vi "Obtain Semaphore Reference.vi"(4 "error in (no error)":errorcluster, 5 "create if not found (T)":bool=TRUE, 6 "size (1)":i32=1, 7 "name (unnamed)":string) -> (0 "error out":errorcluster, 1 "created new":bool, 3 "semaphore":T1)   [LabVIEW 2020]
doc: "Obtains a reference to an existing semaphore or creates a new semaphore and returns a reference to that semaphore."
uses:
  Semaphore Refnum Core.ctl
  GetNamedSemaphorePrefix.vi
panel:
  in  "Size Mismatch\nWarning":string="<err>You specified a named semaphore that already exists, but the existing semaphore has a different size than the one you specified. LabVIEW returned a reference to the existing semaphore but did not resize the semaphore."
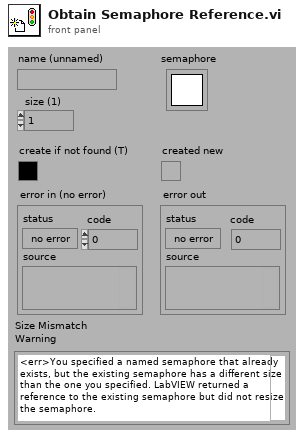
[diagram p1: front panel]
types:
  T1 = typedef "Semaphore RefNum" = refnum<k1>
  T2 = typedef "Semaphore Refnum Core.ctl" = refnum<k1>
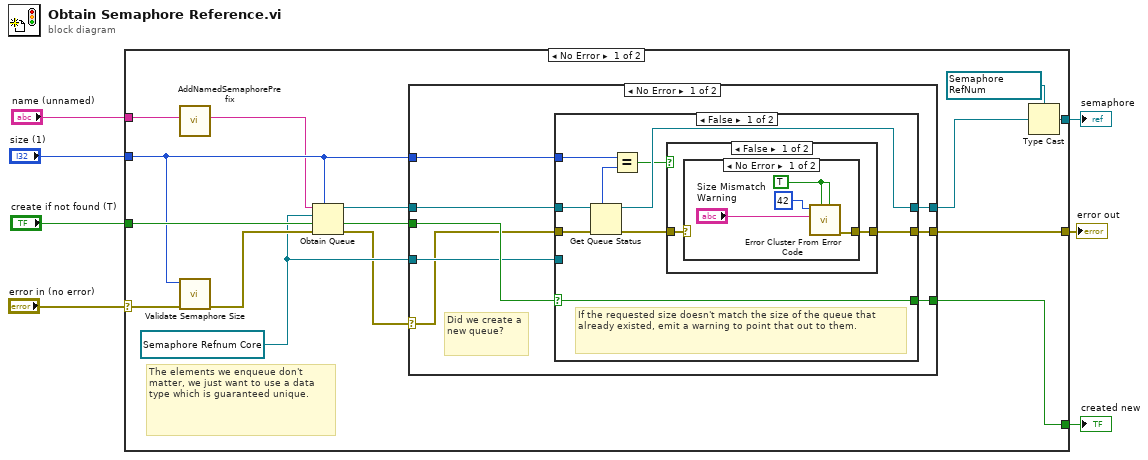
[diagram p0: block diagram]
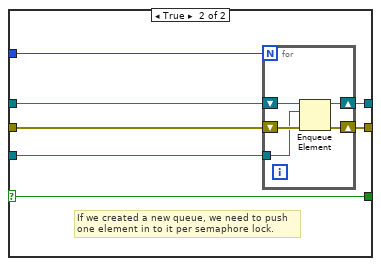
[diagram p4: hidden frame]
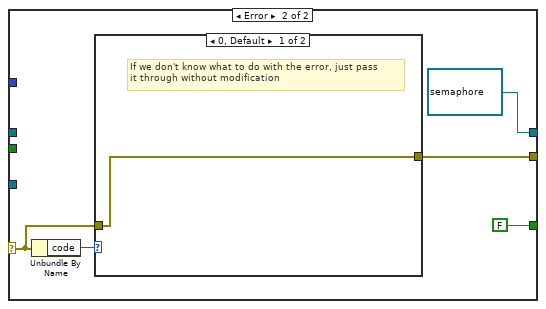
[diagram p5: hidden frame]
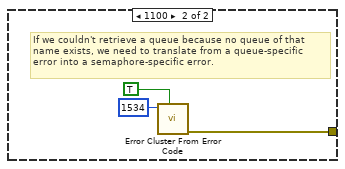
[diagram p6: hidden frame]
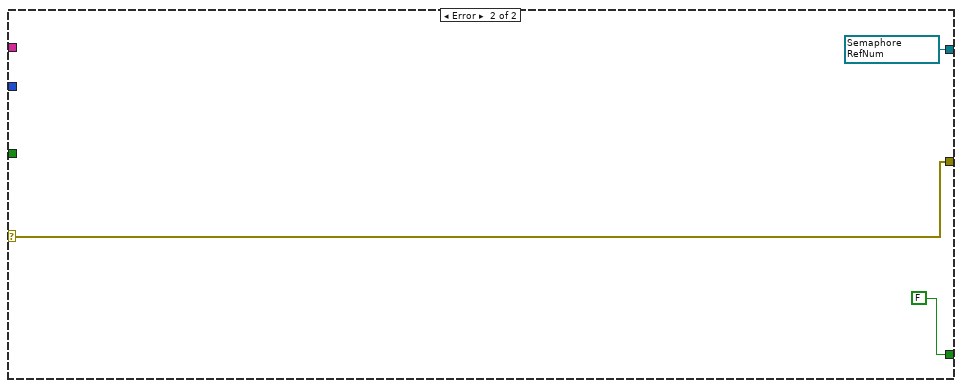
[diagram p7: hidden frame]
diagram:
  n1 = case shown="No Error" "error in (no error)" {
    selector: "error in (no error)" -> [w13 w70]
    tunnel: "create if not found (T)" -> [w21 _]
    tunnel: "name (unnamed)" -> [w9 _]
    tunnel: [w20 w69] -> w6
    tunnel: [w17 w70] -> w5
    tunnel: [w10 FALSE ("created new?")] -> w4
    tunnel: "size (1)" -> [w15 _]
    frame No Error {
      w14 = T2 refnum items=["Semaphore Core"] ("semaphore")
      w19 = T1 refnum items=["semaphore"] ("semaphore")
      # "The elements we enqueue don't matter, we just want to use a data type which is guaranteed unique."
      n2 = call "AddNamedSemaphorePrefix.vi"("String In"=w9) -> ("String Out"=w8:string)  [unwired: 10 out]
      n3 = call "Validate Semaphore Size.vi"("error in (no error)"=w13, "size (1)"=w15) -> ("error out"=w16:errorcluster)  [unwired: 5 out]
      n4 = Obtain Queue(max queue size (-1, unlimited)=w15, name (unnamed)=w8, element data type=w14, create if not found? (T)=w21, error in (no error)=w16) -> (queue out=w22:refnum<queue>, created new?=w11:bool, error out=w12:errorcluster)
      n5 = case shown="No Error" w12 {
        selector: w12 -> [w24 w62]
        tunnel: w22 -> [w30 _]
        tunnel: [w29 w60] -> w18
        tunnel: [w28 w61] -> w17
        tunnel: w11 -> [w27 _]
        tunnel: w15 -> [w26 _]
        tunnel: w14 -> [w25 _]
        tunnel: [w23 FALSE] -> w10
        frame No Error {
          # "Did we create a new queue?"
          n6 = case shown="False" w27 {
            selector: w27 -> [w31 w48]
            tunnel: w30 -> [w38 w54]
            tunnel: w24 -> [w39 w53]
            tunnel: w25 -> [_ w52]
            tunnel: w26 -> [w36 w51]
            tunnel: [w33 w50] -> w29
            tunnel: [w34 w49] -> w28
            tunnel: [w31 w48] -> w23
            frame False {
              # "If the requested size doesn't match the size of the queue that already existed, emit a warning to point that out to them."
              n7 = Get Queue Status(queue=w38, error in (no error)=w39) -> (queue out=w33:refnum<queue>, max queue size=w37:i32, error out=w35:errorcluster)  [unwired: 6 out]
              n8 = Equal?(x=w36, y=w37) -> (x = y?=w32:bool)
              n9 = case shown="False" w32 {
                tunnel: w35 -> [w41 w47]
                tunnel: [w40 w47] -> w34
                frame False {
                  n10 = case shown="No Error" w41 {
                    selector: w41 -> [_ w46]
                    tunnel: [w45 w46] -> w40
                    frame No Error {
                      w42 = TRUE ("show call chain? (False)")
                      n11 = call "Error Cluster From Error Code.vi"("is warning? (False)"=w42, "show call chain? (False)"=w42, "error message (\"\")"="Size Mismatch\nWarning", "error code (0)"=42) -> ("error out"=w45:errorcluster)  [unwired: 1 in, 4 out]
                    }
                    frame Error {
                    }
                  }
                }
                frame True {
                }
              }
            }
            frame True {
              # "If we created a new queue, we need to push one element in to it per semaphore lock."
              n12 = for {
                N: w51 -> [_]
                tunnel: w52 -> [w57]
                shift-right: [w56] -> w49
                shift-left: w53 -> [w58]
                shift-right: [w55] -> w50
                shift-left: w54 -> [w59]
                n13 = Enqueue Element(queue=w59, element=w57, error in (no error)=w58) -> (queue out=w55:refnum<queue>, error out=w56:errorcluster)  [unwired: 2 out]
              }
            }
          }
        }
        frame Error {
          w60 = refnum<queue> refnum items=["Semaphore Core"] ("queue out")
          n14 = Unbundle By Name(w62) -> ("code"=w63:i32)
          n15 = case shown="0, Default" w63 {
            tunnel: w62 -> [w65 _]
            tunnel: [w65 w68] -> w61
            frame 0, Default {
              # "If we don't know what to do with the error, just pass\nit through without modification"
            }
            frame 1100 {
              # "If we couldn't retrieve a queue because no queue of that\nname exists, we need to translate from a queue-specific\nerror into a semaphore-specific error."
              n16 = call "Error Cluster From Error Code.vi"("show call chain? (False)"=TRUE, "error code (0)"=1534) -> ("error out"=w68:errorcluster)  [unwired: 1 in, 6 out]
            }
          }
        }
      }
      n17 = Type Cast(type=w19, x=w18) -> (*(type *) &x=w20:T1)
    }
    frame Error {
      w69 = T1 refnum items=["semaphore"] ("semaphore")
    }
  }
  "error out" <- w5
  "semaphore" <- w6
  "created new" <- w4
